vi "error.vi"() -> ()   [LabVIEW 2017]
uses:
  <vilib>/Analysis/baseanly.llb/Mean (DBL).vi
  <vilib>/Analysis/NI_AALBase.lvlib
panel:
  out "sum":dbl
  out "size(s)":i32
  out "deviation":dbl
  out "x/y":dbl
  in  "numeric array":dbl[](array[numeric])
  out "mean":dbl format="%0.2f"
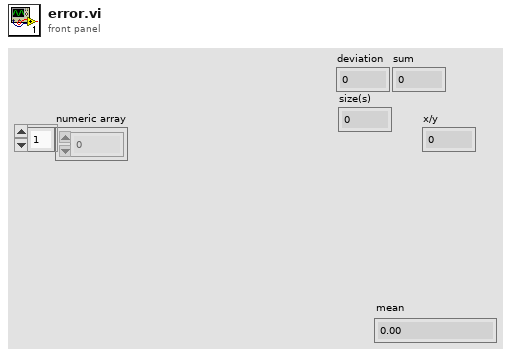
[diagram p1: front panel]
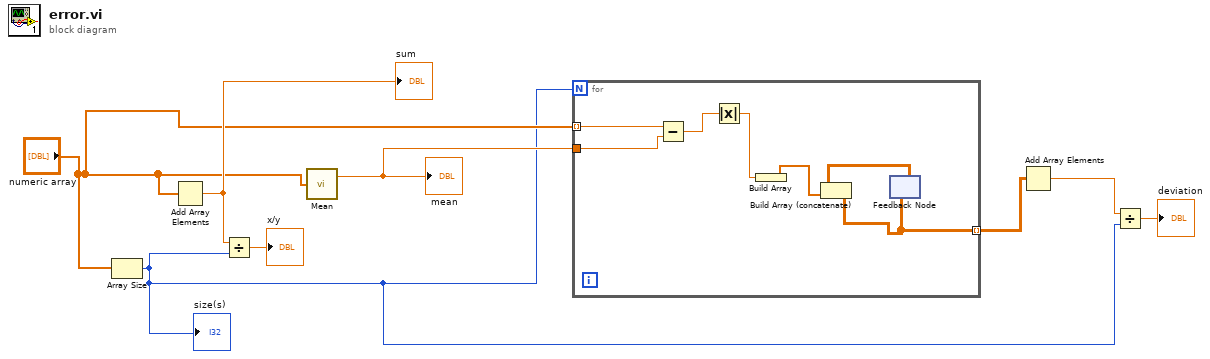
[diagram p0: block diagram]
diagram:
  n1 = Array Size(array="numeric array") -> (size(s)=w2:i32)
  "size(s)" <- w2
  n2 = Add Array Elements(numeric array="numeric array") -> (sum=w8:dbl)
  "sum" <- w8
  n3 = Divide(x=w8, y=w2) -> (x/y=→"x/y":dbl)
  n4 = call-poly <vilib>:"Mean.vi"("X"="numeric array") -> ("mean"=w6:dbl)  [unwired: 1 out]
  "mean" <- w6
  n5 = for {
    N: w2 -> [_]
    tunnel: w6 -> [w15]
    tunnel: "numeric array" -> [w14] mode=indexing
    tunnel: [w11] -> w5 mode=indexing
    n6 = Subtract(x=w14, y=w15) -> (x-y=w10:dbl)
    n7 = Absolute Value(x=w10) -> (abs(x)=w9:dbl)
    n8 = Build Array(w9) -> (w13:dbl[])
    n9 = feedback #1() -> (w12:dbl[][])  [unwired: 1 in]
    n10 = Build Array (concatenate)(w12, w13) -> (w11:dbl[][])
    n11 = feedback-in #1(w11) -> ()
  }
  n12 = Add Array Elements(numeric array=w5) -> (sum=w3:dbl)
  n13 = Divide(x=w3, y=w2) -> (x/y=→"deviation":dbl)
